vi "Read Config.vi"() -> ()   [LabVIEW 2020]
uses:
  PLCMonitor/Read Config.ctl
  PLCMonitor/DataType.ctl
panel:
  in  "Read Config 2":T1={"Start address"="", "length"=1, "type"=enum."Invalid Type"}
  in  "Read Config":T2={"Start address"="", "length"=1, "Data type"=enum."Invalid Type"}
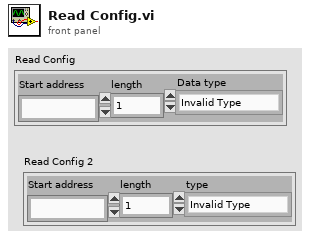
[diagram p1: front panel]
types:
  T1 = cluster{"Start address":string, "length":u16, "type":enum8{"Invalid Type", "Void", "I8", "I16", "I32", "I64", "U8", "U16", "U32", "U64", "Single Float", "Double Float", "Extended Float", "Single Complex", "Double Complex", "Extended Complex", "Enum U8", "Enum U16", "Enum U32", "Enum U64", "Single Float With Unit", "Double Float With Unit", "Extended Float With Unit", "Single Complex with Unit", "Double Complex with Unit", "Extended Complex with Unit", "Boolean", "String", "Path", "Picture", "Tag", "Array", "Cluster", "Variant", "LV Variant", "Waveform", "Timestamp", "Digital Waveform", "Digital Data", "ExpressData", "Refnum", "External Data", "VI", "Poly VI", "LabVIEW Class Instance", "Fixed Point", "Set Collection", "Map Collection"}}
  T2 = typedef "Read Config.ctl" = cluster{"Start address":string, "length":u16, "Data type":T3}
  T3 = typedef "DataType.ctl" = enum8{"Invalid Type", "Void", "I16", "I32", "I64", "U16", "U32", "U64", "Single Float", "Double Float", "Boolean", "String"}
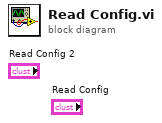
[diagram p0: block diagram]
diagram:
